vi "C4Dev_getFeatureType.vi"(0 "c4dev in":refnum<k24>, 7 "name in":string, 11 "error in":errorcluster) -> (4 "c4dev out":refnum<k24>, 8 "type out":i64(ring) items=["UNKNOWN", "INTEGER", "FLOAT", "STRING", "ENUMERATION", "COMMAND", "BOOLEAN"], 15 "error out":errorcluster)   [LabVIEW 2015, in "libC4HdlLV.lvlib"]
uses:
  libC4HdlLV.lvlib
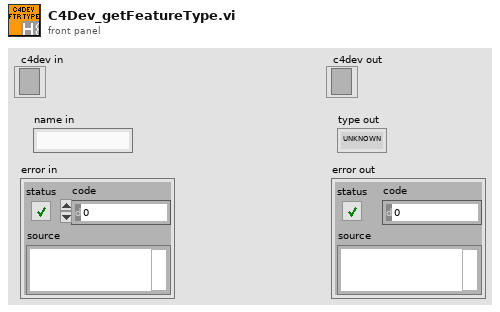
[diagram p1: front panel]
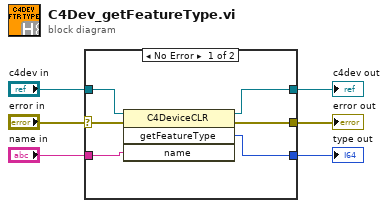
[diagram p0: block diagram]
diagram:
  n1 = case shown="No Error" "error in" {
    selector: "error in" -> [w9 w14]
    tunnel: [w8 w14] -> w5
    tunnel: "c4dev in" -> [w12 w13]
    tunnel: [w10 w13] -> w3
    tunnel: [w11 _] -> w2
    tunnel: "name in" -> [w7 _]
    frame No Error {
      n2 = invoke class="C4DeviceCLR" method="getFeatureType"(reference=w12, error in=w9, "name"=w7) -> (reference out=w10:refnum<k24>, error out=w8:errorcluster, "getFeatureType"=w11:i64)  [unwired: 1 in, 1 out]
    }
    frame Error {
    }
  }
  "error out" <- w5
  "c4dev out" <- w3
  "type out" <- w2
